vi "Holding Var.vi"() -> ()   [LabVIEW 2016]
panel:
  in  "控制模式":enum16{"手动", "自动"}(ring)
  in  "关闭时间（H）":u16=6
  in  "开启时间（H）":u16=20
  in  "总开关":bool
  in  "CODCr":T1={"水样测试"={"参数输入"={"采样模式"=enum."自动采样", "采样点数"=3, "变异系数设定值"=0.1, "重新取值百分比"=0.5, "偏差模式"=enum."相对偏差", "相对偏差百分比"=0.5, "绝对偏差值"=0.0}, "采样值"=[], "启用"=FALSE}, "零点核查"={"参数输入"={"采样模式"=enum."自动采样", "采样点数"=3, "变异系数设定值"=0.1, "重新取值百分比"=0.5, "偏差模式"=enum."相对偏差", "相对偏差百分比"=0.5, "绝对偏差值"=0.0}, "采样值"=[], "启用"=FALSE}, "跨度核查"={"参数输入"={"采样模式"=enum."自动采样", "采样点数"=3, "变异系数设定值"=0.1, "重新取值百分比"=0.5, "偏差模式"=enum."相对偏差", "相对偏差百分比"=0.5, "绝对偏差值"=0.0}, "采样值"=[], "启用"=FALSE}}
  in  "CODMn":T1={"水样测试"={"参数输入"={"采样模式"=enum."自动采样", "采样点数"=3, "变异系数设定值"=0.1, "重新取值百分比"=0.5, "偏差模式"=enum."相对偏差", "相对偏差百分比"=0.5, "绝对偏差值"=0.0}, "采样值"=[], "启用"=FALSE}, "零点核查"={"参数输入"={"采样模式"=enum."自动采样", "采样点数"=3, "变异系数设定值"=0.1, "重新取值百分比"=0.5, "偏差模式"=enum."相对偏差", "相对偏差百分比"=0.5, "绝对偏差值"=0.0}, "采样值"=[], "启用"=FALSE}, "跨度核查"={"参数输入"={"采样模式"=enum."自动采样", "采样点数"=3, "变异系数设定值"=0.1, "重新取值百分比"=0.5, "偏差模式"=enum."相对偏差", "相对偏差百分比"=0.5, "绝对偏差值"=0.0}, "采样值"=[], "启用"=FALSE}}
  in  "TN":T1={"水样测试"={"参数输入"={"采样模式"=enum."自动采样", "采样点数"=3, "变异系数设定值"=0.1, "重新取值百分比"=0.5, "偏差模式"=enum."相对偏差", "相对偏差百分比"=0.5, "绝对偏差值"=0.0}, "采样值"=[], "启用"=FALSE}, "零点核查"={"参数输入"={"采样模式"=enum."自动采样", "采样点数"=3, "变异系数设定值"=0.1, "重新取值百分比"=0.5, "偏差模式"=enum."相对偏差", "相对偏差百分比"=0.5, "绝对偏差值"=0.0}, "采样值"=[], "启用"=FALSE}, "跨度核查"={"参数输入"={"采样模式"=enum."自动采样", "采样点数"=3, "变异系数设定值"=0.1, "重新取值百分比"=0.5, "偏差模式"=enum."相对偏差", "相对偏差百分比"=0.5, "绝对偏差值"=0.0}, "采样值"=[], "启用"=FALSE}}
  in  "TP":T1={"水样测试"={"参数输入"={"采样模式"=enum."自动采样", "采样点数"=3, "变异系数设定值"=0.1, "重新取值百分比"=0.5, "偏差模式"=enum."相对偏差", "相对偏差百分比"=0.5, "绝对偏差值"=0.0}, "采样值"=[], "启用"=FALSE}, "零点核查"={"参数输入"={"采样模式"=enum."自动采样", "采样点数"=3, "变异系数设定值"=0.1, "重新取值百分比"=0.5, "偏差模式"=enum."相对偏差", "相对偏差百分比"=0.5, "绝对偏差值"=0.0}, "采样值"=[], "启用"=FALSE}, "跨度核查"={"参数输入"={"采样模式"=enum."自动采样", "采样点数"=3, "变异系数设定值"=0.1, "重新取值百分比"=0.5, "偏差模式"=enum."相对偏差", "相对偏差百分比"=0.5, "绝对偏差值"=0.0}, "采样值"=[], "启用"=FALSE}}
  in  "NH3N":T1={"水样测试"={"参数输入"={"采样模式"=enum."自动采样", "采样点数"=3, "变异系数设定值"=0.1, "重新取值百分比"=0.5, "偏差模式"=enum."相对偏差", "相对偏差百分比"=0.5, "绝对偏差值"=0.0}, "采样值"=[], "启用"=FALSE}, "零点核查"={"参数输入"={"采样模式"=enum."自动采样", "采样点数"=3, "变异系数设定值"=0.1, "重新取值百分比"=0.5, "偏差模式"=enum."相对偏差", "相对偏差百分比"=0.5, "绝对偏差值"=0.0}, "采样值"=[], "启用"=FALSE}, "跨度核查"={"参数输入"={"采样模式"=enum."自动采样", "采样点数"=3, "变异系数设定值"=0.1, "重新取值百分比"=0.5, "偏差模式"=enum."相对偏差", "相对偏差百分比"=0.5, "绝对偏差值"=0.0}, "采样值"=[], "启用"=FALSE}}
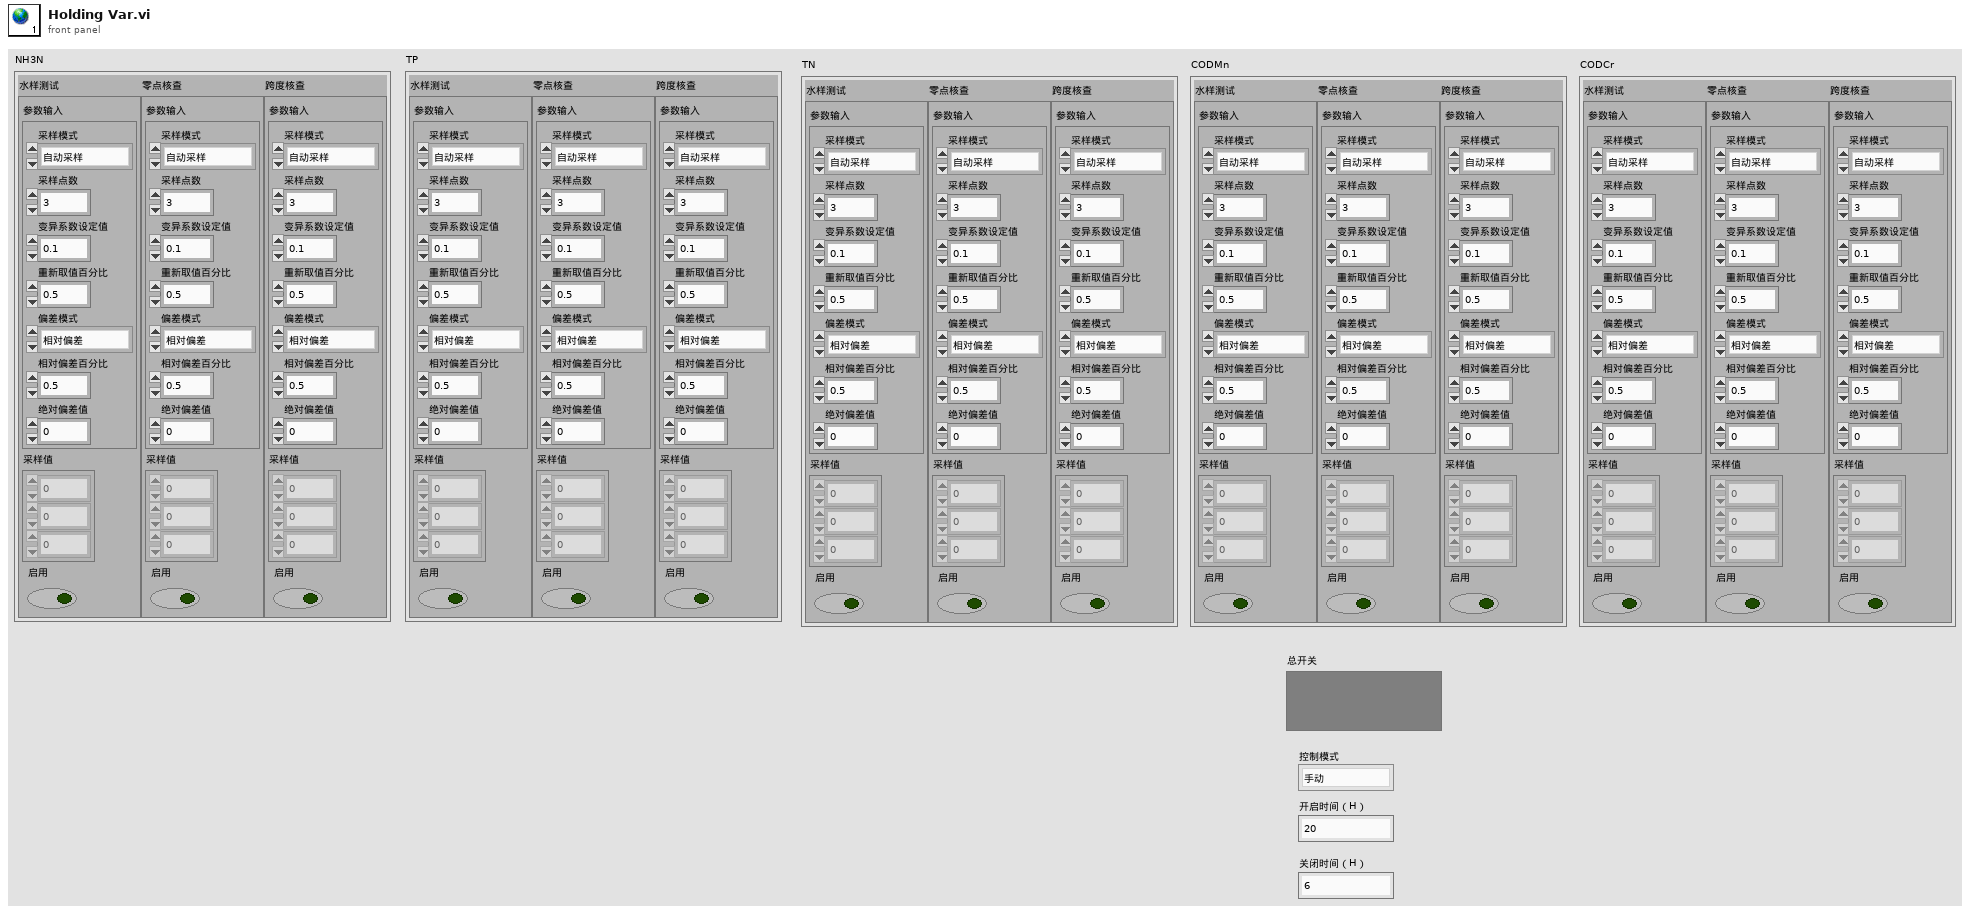
[diagram p1: front panel]
types:
  T1 = cluster{"水样测试":cluster{"参数输入":cluster{"采样模式":enum16{"自动采样", "手动采样"}, "采样点数":i32, "变异系数设定值":dbl, "重新取值百分比":dbl, "偏差模式":enum16{"相对偏差", "绝对偏差"}, "相对偏差百分比":dbl, "绝对偏差值":dbl}, "采样值":dbl[], "启用":bool}, "零点核查":cluster{"参数输入":cluster{"采样模式":enum16{"自动采样", "手动采样"}, "采样点数":i32, "变异系数设定值":dbl, "重新取值百分比":dbl, "偏差模式":enum16{"相对偏差", "绝对偏差"}, "相对偏差百分比":dbl, "绝对偏差值":dbl}, "采样值":dbl[], "启用":bool}, "跨度核查":cluster{"参数输入":cluster{"采样模式":enum16{"自动采样", "手动采样"}, "采样点数":i32, "变异系数设定值":dbl, "重新取值百分比":dbl, "偏差模式":enum16{"相对偏差", "绝对偏差"}, "相对偏差百分比":dbl, "绝对偏差值":dbl}, "采样值":dbl[], "启用":bool}}
diagram:
